vi "BootstrapProcessingLoop.vi"(8 "error in (no error)":errorcluster, 11 "navX in":refnum<class "navX.lvclass">) -> (0 "error out":errorcluster, 3 "navX out":refnum<class "navX.lvclass">)   [LabVIEW 2015, in "navX Library v3.lvlib" / "navX.lvclass"]
uses:
  navX.lvclass
  navX.lvclass/navX.ctl
  navX - Interface/navX - Interface.lvclass
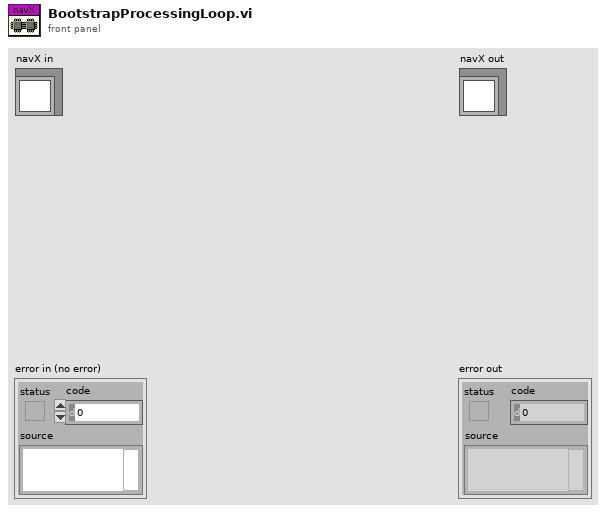
[diagram p1: front panel]
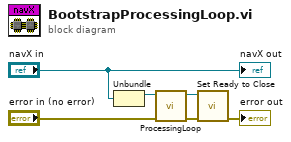
[diagram p0: block diagram]
diagram:
  n1 = Unbundle("navX in") -> (w4:refnum<class "navX - Interface.lvclass">)  [unwired: 1 out]
  n2 = call-dynamic "ProcessingLoop.vi"("error in (no error)"="error in (no error)", "navX - Interface in"=w4) -> ("error out"=w2:errorcluster, "navX - Interface out"=w3:refnum<class "navX - Interface.lvclass">)  [unwired: 8 in]
  n3 = call "Set Ready to Close.vi"("error in (no error)"=w2, "navX - Interface in"=w3) -> ("error out"=→"error out":errorcluster)  [unwired: 8 in, 1 out]
  "navX out" <- "navX in"
